vi "Main Tclk.vi"() -> ()   [LabVIEW 2018] (continued)
                        n2265 = local read "BD2 high limit array"() -> (w8137:sgl[])
                        n2266 = local read "Milling I high limit array"() -> (w8134:sgl[])
                        n2267 = local read "BD1 low limit array"() -> (w8112:sgl[])
                        n2268 = local read "BD2 low limit array"() -> (w8138:sgl[])
                        n2269 = local read "Milling I low limit array"() -> (w8133:sgl[])
                        n2270 = Build Array (concatenate)(w8147, w8123) -> (w8146:sgl[])
                        n2271 = In Range and Coerce(upper limit=w8123, x=w8100, lower limit=w8122) -> (In Range?=w8125:bool)  [unwired: 1 out]
                        n2272 = Build Array (concatenate)(w8148, w8122) -> (w8149:sgl[])
                        n2273 = Build Array (concatenate)(w8106, w8105) -> (w8113:sgl[])
                        n2274 = In Range and Coerce(upper limit=w8105, x=w8103, lower limit=w8104) -> (In Range?=w8109:bool)  [unwired: 1 out]
                        n2275 = Build Array (concatenate)(w8112, w8104) -> (w8111:sgl[])
                        n2276 = Build Array (concatenate)(w8137, w8119) -> (w8136:sgl[])
                        n2277 = In Range and Coerce(upper limit=w8119, x=w8102, lower limit=w8118) -> (In Range?=w8121:bool)  [unwired: 1 out]
                        n2278 = Build Array (concatenate)(w8138, w8118) -> (w8139:sgl[])
                        n2279 = Build Array (concatenate)(w8134, w8115) -> (w8135:sgl[])
                        n2280 = In Range and Coerce(upper limit=w8115, x=w8101, lower limit=w8114) -> (In Range?=w8117:bool)  [unwired: 1 out]
                        n2281 = Build Array (concatenate)(w8133, w8114) -> (w8132:sgl[])
                        n2282 = Not(x=w8125) -> (.not. x?=w8124:bool)
                        n2283 = Not(x=w8109) -> (.not. x?=w8110:bool)
                        n2284 = Not(x=w8121) -> (.not. x?=w8120:bool)
                        n2285 = Not(x=w8117) -> (.not. x?=w8116:bool)
                        n2286 = local write "Specimen I high limit array"(w8146) -> ()
                        n2287 = local write "Specimen I low limit array"(w8149) -> ()
                        n2288 = local write "BD1 high limit array"(w8113) -> ()
                        n2289 = local write "BD2 high limit array"(w8136) -> ()
                        n2290 = local write "Milling I high limit array"(w8135) -> ()
                        n2291 = local write "BD1 low limit array"(w8111) -> ()
                        n2292 = local write "BD2 low limit array"(w8139) -> ()
                        n2293 = local write "Milling I low limit array"(w8132) -> ()
                        n2294 = local write "Specimen I out of bound"(w8124) -> ()
                        n2295 = local write "BD1 out of bound"(w8110) -> ()
                        n2296 = local write "BD2 out of bound"(w8120) -> ()
                        n2297 = local write "Milling I out of bound"(w8116) -> ()
                      }
                      frame 2 {
                        n2298 = local read "Specimen I array"() -> (w8208:sgl[])
                        n2299 = local read "Specimen I (nA)"() -> (w8156:sgl)
                        n2300 = local read "Beam Dump 1 array"() -> (w8195:sgl[])
                        n2301 = local read "Beam Dump 1 (nA)"() -> (w8159:sgl)
                        n2302 = local read "Beam Dump 2 (nA)"() -> (w8165:sgl)
                        n2303 = local read "Milling I array"() -> (w8185:sgl[])
                        n2304 = local read "Milling I (nA)"() -> (w8164:sgl)
                        n2305 = call "Auto limits.vi"("Minimum half range"=0.5, "# of interquartile range or stdev"=6.0 ("# of sigma"), "Length"=100, "Input array"=w8208) -> ("Low limit"=w8206:dbl, "High limit"=w8207:dbl)  [unwired: 5 in, 1 out]
                        n2306 = call "Auto limits.vi"("Minimum half range"=0.5, "# of interquartile range or stdev"=6.0 ("# of sigma"), "Length"=100, "Input array"=w8195) -> ("Low limit"=w8197:dbl, "High limit"=w8196:dbl)  [unwired: 5 in, 1 out]
                        n2307 = call "Auto limits.vi"("Minimum half range"=0.5, "# of interquartile range or stdev"=6.0 ("# of sigma"), "Length"=100, "Input array"=w8185) -> ("Low limit"=w8187:dbl, "High limit"=w8186:dbl)  [unwired: 5 in, 1 out]
                        n2308 = To Single Precision Float(number=w8207) -> (single precision float=w8158:sgl)
                        n2309 = To Single Precision Float(number=w8206) -> (single precision float=w8157:sgl)
                        n2310 = To Single Precision Float(number=w8196) -> (single precision float=w8161:sgl)
                        n2311 = To Single Precision Float(number=w8197) -> (single precision float=w8160:sgl)
                        n2312 = To Single Precision Float(number=w8167) -> (single precision float=w8169:sgl)
                        n2313 = To Single Precision Float(number=w8166) -> (single precision float=w8168:sgl)
                        n2314 = To Single Precision Float(number=w8186) -> (single precision float=w8163:sgl)
                        n2315 = To Single Precision Float(number=w8187) -> (single precision float=w8162:sgl)
                        n2316 = local read "Specimen I high limit array"() -> (w8203:sgl[])
                        n2317 = local read "Specimen I low limit array"() -> (w8204:sgl[])
                        n2318 = local read "BD1 high limit array"() -> (w8200:sgl[])
                        n2319 = local read "BD2 high limit array"() -> (w8173:sgl[])
                        n2320 = local read "Milling I high limit array"() -> (w8190:sgl[])
                        n2321 = local read "BD1 low limit array"() -> (w8199:sgl[])
                        n2322 = local read "BD2 low limit array"() -> (w8174:sgl[])
                        n2323 = local read "Milling I low limit array"() -> (w8189:sgl[])
                        n2324 = Build Array (concatenate)(w8203, w8158) -> (w8202:sgl[])
                        n2325 = In Range and Coerce(upper limit=w8158, x=w8156, lower limit=w8157) -> (In Range?=w8181:bool)  [unwired: 1 out]
                        n2326 = Build Array (concatenate)(w8204, w8157) -> (w8205:sgl[])
                        n2327 = Build Array (concatenate)(w8200, w8161) -> (w8201:sgl[])
                        n2328 = In Range and Coerce(upper limit=w8161, x=w8159, lower limit=w8160) -> (In Range?=w8178:bool)  [unwired: 1 out]
                        n2329 = Build Array (concatenate)(w8199, w8160) -> (w8198:sgl[])
                        n2330 = Build Array (concatenate)(w8173, w8169) -> (w8172:sgl[])
                        n2331 = In Range and Coerce(upper limit=w8169, x=w8165, lower limit=w8168) -> (In Range?=w8171:bool)  [unwired: 1 out]
                        n2332 = Build Array (concatenate)(w8174, w8168) -> (w8175:sgl[])
                        n2333 = Build Array (concatenate)(w8190, w8163) -> (w8191:sgl[])
                        n2334 = In Range and Coerce(upper limit=w8163, x=w8164, lower limit=w8162) -> (In Range?=w8177:bool)  [unwired: 1 out]
                        n2335 = Build Array (concatenate)(w8189, w8162) -> (w8188:sgl[])
                        n2336 = Not(x=w8181) -> (.not. x?=w8180:bool)
                        n2337 = Not(x=w8178) -> (.not. x?=w8179:bool)
                        n2338 = Not(x=w8171) -> (.not. x?=w8170:bool)
                        n2339 = Not(x=w8177) -> (.not. x?=w8176:bool)
                        n2340 = local write "Specimen I high limit array"(w8202) -> ()
                        n2341 = local write "Specimen I low limit array"(w8205) -> ()
                        n2342 = local write "BD1 high limit array"(w8201) -> ()
                        n2343 = local write "BD2 high limit array"(w8172) -> ()
                        n2344 = local write "Milling I high limit array"(w8191) -> ()
                        n2345 = local write "BD1 low limit array"(w8198) -> ()
                        n2346 = local write "BD2 low limit array"(w8175) -> ()
                        n2347 = local write "Milling I low limit array"(w8188) -> ()
                        n2348 = local write "Specimen I out of bound"(w8180) -> ()
                        n2349 = local write "BD1 out of bound"(w8179) -> ()
                        n2350 = local write "BD2 out of bound"(w8170) -> ()
                        n2351 = local write "Milling I out of bound"(w8176) -> ()
                      }
                      frame 3 {
                        n2352 = local read "Specimen I array"() -> (w8267:sgl[])
                        n2353 = local read "Specimen I (nA)"() -> (w8241:sgl)
                        n2354 = local read "Beam Dump 1 array"() -> (w8254:sgl[])
                        n2355 = local read "Beam Dump 1 (nA)"() -> (w8219:sgl)
                        n2356 = local read "Beam Dump 2 array"() -> (w8251:sgl[])
                        n2357 = local read "Beam Dump 2 (nA)"() -> (w8237:sgl)
                        n2358 = local read "Milling I (nA)"() -> (w8224:sgl)
                        n2359 = expression code="X*6"(w8212) -> (w8218:sgl)
                        n2360 = expression code="X*0.5"(w8212) -> (w8217:sgl)
                        n2361 = expression code="X*6"(w8212) -> (w8214:sgl)
                        n2362 = expression code="X*0.5"(w8212) -> (w8213:sgl)
                        n2363 = expression code="X*3"(w8212) -> (w8216:sgl)
                        n2364 = expression code="X*0.2"(w8212) -> (w8215:sgl)
                        n2365 = call "Auto limits.vi"("Minimum half range"=w8217, "# of interquartile range or stdev"=w8218, "Length"=100, "Input array"=w8267) -> ("Low limit"=w8265:dbl, "High limit"=w8266:dbl)  [unwired: 5 in, 1 out]
                        n2366 = call "Auto limits.vi"("Minimum half range"=w8213, "# of interquartile range or stdev"=w8214, "Length"=100, "Input array"=w8254) -> ("Low limit"=w8256:dbl, "High limit"=w8255:dbl)  [unwired: 5 in, 1 out]
                        n2367 = call "Auto limits.vi"("Minimum half range"=w8215, "# of interquartile range or stdev"=w8216, "Length"=100, "Input array"=w8251) -> ("Low limit"=w8249:dbl, "High limit"=w8250:dbl)  [unwired: 5 in, 1 out]
                        n2368 = To Single Precision Float(number=w8266) -> (single precision float=w8243:sgl)
                        n2369 = To Single Precision Float(number=w8265) -> (single precision float=w8242:sgl)
                        n2370 = To Single Precision Float(number=w8255) -> (single precision float=w8221:sgl)
                        n2371 = To Single Precision Float(number=w8256) -> (single precision float=w8220:sgl)
                        n2372 = To Single Precision Float(number=w8250) -> (single precision float=w8239:sgl)
                        n2373 = To Single Precision Float(number=w8249) -> (single precision float=w8238:sgl)
                        n2374 = To Single Precision Float(number=w8231) -> (single precision float=w8226:sgl)
                        n2375 = To Single Precision Float(number=w8230) -> (single precision float=w8225:sgl)
                        n2376 = local read "Specimen I high limit array"() -> (w8262:sgl[])
                        n2377 = local read "Specimen I low limit array"() -> (w8263:sgl[])
                        n2378 = local read "BD1 high limit array"() -> (w8259:sgl[])
                        n2379 = local read "BD2 high limit array"() -> (w8246:sgl[])
                        n2380 = local read "BD2 low limit array"() -> (w8247:sgl[])
                        n2381 = local read "Milling I high limit array"() -> (w8235:sgl[])
                        n2382 = local read "BD1 low limit array"() -> (w8258:sgl[])
                        n2383 = local read "Milling I low limit array"() -> (w8234:sgl[])
                        n2384 = Build Array (concatenate)(w8247, w8238) -> (w8248:sgl[])
                        n2385 = Build Array (concatenate)(w8262, w8243) -> (w8261:sgl[])
                        n2386 = In Range and Coerce(upper limit=w8243, x=w8241, lower limit=w8242) -> (In Range?=w8244:bool)  [unwired: 1 out]
                        n2387 = Build Array (concatenate)(w8263, w8242) -> (w8264:sgl[])
                        n2388 = Build Array (concatenate)(w8259, w8221) -> (w8260:sgl[])
                        n2389 = In Range and Coerce(upper limit=w8221, x=w8219, lower limit=w8220) -> (In Range?=w8222:bool)  [unwired: 1 out]
                        n2390 = Build Array (concatenate)(w8258, w8220) -> (w8257:sgl[])
                        n2391 = Build Array (concatenate)(w8246, w8239) -> (w8245:sgl[])
                        n2392 = In Range and Coerce(upper limit=w8239, x=w8237, lower limit=w8238) -> (In Range?=w8240:bool)  [unwired: 1 out]
                        n2393 = Build Array (concatenate)(w8235, w8226) -> (w8236:sgl[])
                        n2394 = In Range and Coerce(upper limit=w8226, x=w8224, lower limit=w8225) -> (In Range?=w8232:bool)  [unwired: 1 out]
                        n2395 = Build Array (concatenate)(w8234, w8225) -> (w8233:sgl[])
                        n2396 = Not(x=w8244) -> (.not. x?=w8229:bool)
                        n2397 = Not(x=w8222) -> (.not. x?=w8223:bool)
                        n2398 = Not(x=w8240) -> (.not. x?=w8228:bool)
                        n2399 = Not(x=w8232) -> (.not. x?=w8227:bool)
                        n2400 = local write "Specimen I high limit array"(w8261) -> ()
                        n2401 = local write "Specimen I low limit array"(w8264) -> ()
                        n2402 = local write "BD1 high limit array"(w8260) -> ()
                        n2403 = local write "BD2 high limit array"(w8245) -> ()
                        n2404 = local write "BD2 low limit array"(w8248) -> ()
                        n2405 = local write "Milling I high limit array"(w8236) -> ()
                        n2406 = local write "BD1 low limit array"(w8257) -> ()
                        n2407 = local write "Milling I low limit array"(w8233) -> ()
                        n2408 = local write "Specimen I out of bound"(w8229) -> ()
                        n2409 = local write "BD1 out of bound"(w8223) -> ()
                        n2410 = local write "BD2 out of bound"(w8228) -> ()
                        n2411 = local write "Milling I out of bound"(w8227) -> ()
                      }
                      frame 100, Default {
                        n2412 = local read "Specimen I array"() -> (w8313:sgl[])
                        n2413 = local read "Beam Dump 1 array"() -> (w8296:sgl[])
                        n2414 = local read "Beam Dump 2 array"() -> (w8289:sgl[])
                        n2415 = local read "Milling I array"() -> (w8272:sgl[])
                        n2416 = call "Auto limits.vi"("Minimum half range"=0.5, "# of interquartile range or stdev"=6.0 ("# of sigma"), "Length"=100, "Input array"=w8313) -> ("Low limit"=w8311:dbl, "High limit"=w8312:dbl)  [unwired: 5 in, 1 out]
                        n2417 = call "Auto limits.vi"("Minimum half range"=0.5, "# of interquartile range or stdev"=6.0 ("# of sigma"), "Length"=100, "Input array"=w8296) -> ("Low limit"=w8298:dbl, "High limit"=w8297:dbl)  [unwired: 5 in, 1 out]
                        n2418 = call "Auto limits.vi"("Minimum half range"=0.5, "# of interquartile range or stdev"=6.0 ("# of sigma"), "Length"=100, "Input array"=w8289) -> ("Low limit"=w8287:dbl, "High limit"=w8288:dbl)  [unwired: 5 in, 1 out]
                        n2419 = call "Auto limits.vi"("Minimum half range"=0.5, "# of interquartile range or stdev"=6.0 ("# of sigma"), "Length"=100, "Input array"=w8272) -> ("Low limit"=w8274:dbl, "High limit"=w8273:dbl)  [unwired: 5 in, 1 out]
                        n2420 = To Single Precision Float(number=w8312) -> (single precision float=w8306:sgl)
                        n2421 = To Single Precision Float(number=w8311) -> (single precision float=w8305:sgl)
                        n2422 = To Single Precision Float(number=w8297) -> (single precision float=w8303:sgl)
                        n2423 = To Single Precision Float(number=w8298) -> (single precision float=w8304:sgl)
                        n2424 = To Single Precision Float(number=w8288) -> (single precision float=w8282:sgl)
                        n2425 = To Single Precision Float(number=w8287) -> (single precision float=w8281:sgl)
                        n2426 = To Single Precision Float(number=w8273) -> (single precision float=w8279:sgl)
                        n2427 = To Single Precision Float(number=w8274) -> (single precision float=w8280:sgl)
                        n2428 = local read "Specimen I high limit array"() -> (w8308:sgl[])
                        n2429 = local read "Specimen I low limit array"() -> (w8309:sgl[])
                        n2430 = local read "BD1 high limit array"() -> (w8301:sgl[])
                        n2431 = local read "BD2 high limit array"() -> (w8284:sgl[])
                        n2432 = local read "Milling I high limit array"() -> (w8277:sgl[])
                        n2433 = local read "BD1 low limit array"() -> (w8300:sgl[])
                        n2434 = local read "BD2 low limit array"() -> (w8285:sgl[])
                        n2435 = local read "Milling I low limit array"() -> (w8276:sgl[])
                        n2436 = Build Array (concatenate)(w8308, w8306) -> (w8307:sgl[])
                        n2437 = Build Array (concatenate)(w8309, w8305) -> (w8310:sgl[])
                        n2438 = Build Array (concatenate)(w8301, w8303) -> (w8302:sgl[])
                        n2439 = Build Array (concatenate)(w8300, w8304) -> (w8299:sgl[])
                        n2440 = Build Array (concatenate)(w8284, w8282) -> (w8283:sgl[])
                        n2441 = Build Array (concatenate)(w8285, w8281) -> (w8286:sgl[])
                        n2442 = Build Array (concatenate)(w8277, w8279) -> (w8278:sgl[])
                        n2443 = Build Array (concatenate)(w8276, w8280) -> (w8275:sgl[])
                        n2444 = local write "Specimen I high limit array"(w8307) -> ()
                        n2445 = local write "Specimen I low limit array"(w8310) -> ()
                        n2446 = local write "BD1 high limit array"(w8302) -> ()
                        n2447 = local write "BD2 high limit array"(w8283) -> ()
                        n2448 = local write "Milling I high limit array"(w8278) -> ()
                        n2449 = local write "BD1 low limit array"(w8299) -> ()
                        n2450 = local write "BD2 low limit array"(w8286) -> ()
                        n2451 = local write "Milling I low limit array"(w8275) -> ()
                      }
                    }
                  }
                }
                n2452 = local read "Delta X array for stop limit"() -> (w7979:sgl[])
                n2453 = local read "Delta Y array for stop limit"() -> (w7976:sgl[])
                n2454 = local read "X shift (nm/image)"() -> (w7965:sgl)
                n2455 = local read "Y shift (nm/image)"() -> (w7962:sgl)
                n2456 = Absolute Value(x=w7979) -> (abs(x)=w7972:sgl[])
                n2457 = Absolute Value(x=w7976) -> (abs(x)=w7971:sgl[])
                n2458 = local read "Delta X stop limit array"() -> (w7980:sgl[])
                n2459 = local read "Delta Y stop limit array"() -> (w7974:sgl[])
                n2460 = call "Auto limits.vi"("Method"="mean & stdev", "Minimum half range"=10.0 ("# of sigma"), "# of interquartile range or stdev"=6.0 ("# of sigma"), "Length"=10, "Input array"=w7972) -> ("High limit"=w7959:dbl)  [unwired: 4 in, 2 out]
                n2461 = call "Auto limits.vi"("Method"="mean & stdev", "Minimum half range"=10.0 ("# of sigma"), "# of interquartile range or stdev"=6.0 ("# of sigma"), "Length"=100, "Input array"=w7971) -> ("High limit"=w7975:dbl)  [unwired: 4 in, 2 out]
                n2462 = To Single Precision Float(number=w7959) -> (single precision float=w7982:sgl)
                n2463 = To Single Precision Float(number=w7975) -> (single precision float=w7961:sgl)
                n2464 = Absolute Value(x=w7965) -> (abs(x)=w7957:sgl)
                n2465 = Absolute Value(x=w7962) -> (abs(x)=w7958:sgl)
                n2466 = Add(x=w7982, y=w7957) -> (x+y=w7966:sgl)
                n2467 = Add(x=w7961, y=w7958) -> (x+y=w7963:sgl)
                n2468 = Build Array (concatenate)(w7980, w7966) -> (w7981:sgl[])
                n2469 = Build Array (concatenate)(w7974, w7963) -> (w7973:sgl[])
                n2470 = local write "Delta X stop limit array"(w7981) -> ()
                n2471 = local write "Delta Y stop limit array"(w7973) -> ()
              }
              frame #27 {
                n2472 = local read "Pause for reheat"() -> (w8349:bool)
                n2473 = local read "Auto re-engage"() -> (w8348:bool)
                n2474 = case shown="True" w8349 {
                  tunnel: w8348 -> [_ w8358]
                  frame False {
                  }
                  frame True {
                    n2475 = case shown="False" w8358 {
                      frame False {
                        n2476 = stacked-sequence {
                          frame #0 {
                            n2477 = local read "3D FIB-SEM Files"() -> (w8364:path)
                            n2478 = local read "Re-engage Files"() -> (w8367:path)
                            n2479 = Build Path(base path=w8364, name or relative path="LG low res.png " ("command line")) -> (appended path=w8363:path)
                            n2480 = Build Path(base path=w8367, name or relative path="pre.png " ("command line")) -> (appended path=w8362:path)
                            n2481 = Copy(9:TRUE ("run minimized? (F)"), 10:w8362, 11:w8363) -> ()  [unwired: 2 in, 3 out]
                          }
                          frame #1 {
                            n2482 = shared-variable ".\\Zeiss Library.lvlib\\Timestamp"() -> (→"Pre-reheat time":timestamp)  [unwired: 1 in, 1 out]
                            n2483 = local read "Last good FI"() -> (→"Pre-reheat FI":sgl)
                          }
                          frame #2 {
                            n2484 = local read "SEM Scan Parameters"() -> (w8370:T26)
                            n2485 = Unbundle By Name(w8370) -> ("X center (um)"=→"Pre-reheat X center (um)":sgl, "Y center (um)"=→"Pre-reheat Y center (um)":sgl, "Y stig"=w8373:sgl[][])
                            n2486 = local write "Pre-reheat Y stig"(w8373) -> ()
                          }
                        }
                      }
                      frame True {
                      }
                    }
                    n2487 = local write "Mill Manual Pause"(TRUE ("Mill Stop")) -> ()
                    n2488 = property on="Mill Manual Pause" class="Bool (strict)"("DisabledEnum"=T44."Disabled and Grayed Out" ("Disabled")) -> ()  [unwired: 2 in, 2 out]
                  }
                }
                n2489 = local read "Remaining X shift frames"() -> (w8347:u32)
                n2490 = local read "Remaining Y shift frames"() -> (w8342:u32)
                n2491 = Greater Than 0?(x=w8347) -> (x > 0?=w8346:bool)
                n2492 = Greater Than 0?(x=w8342) -> (x > 0?=w8343:bool)
                n2493 = case shown="False" w8346 {
                  tunnel: w8347 -> [_ w8357]
                  tunnel: [u32 0 w8356] -> w8345
                  frame False {
                    n2494 = local write "X shift (nm/image)"(sgl 0.0 ("X shift (nm/image)")) -> ()
                  }
                  frame True {
                    n2495 = Decrement(x=w8357) -> (x-1=w8356:u32)
                  }
                }
                n2496 = case shown="False" w8343 {
                  tunnel: w8342 -> [_ w8353]
                  tunnel: [u32 0 w8352] -> w8344
                  frame False {
                    n2497 = local write "Y shift (nm/image)"(sgl 0.0 ("X shift (nm/image)")) -> ()
                  }
                  frame True {
                    n2498 = Decrement(x=w8353) -> (x-1=w8352:u32)
                  }
                }
                n2499 = local write "Remaining X shift frames"(w8345) -> ()
                n2500 = local write "Remaining Y shift frames"(w8344) -> ()
              }
              frame #28 {
                n2501 = local read "FIB"() -> (w8382:bool)
                n2502 = local read "Alert Settings"() -> (w8380:T36)
                n2503 = local read "Log time array"() -> (w8375:u32[])
                n2504 = case shown="True" w8382 {
                  frame False {
                  }
                  frame True {
                    n2505 = local read "Temp (F)"() -> (w8419:sgl)
                    n2506 = local read "Faraday Cup (nA)"() -> (w8420:sgl)
                    n2507 = local read "Specimen I (nA)"() -> (w8421:sgl)
                    n2508 = local read "Beam Dump 1 (nA)"() -> (w8422:sgl)
                    n2509 = local read "Beam Dump 2 (nA)"() -> (w8413:sgl)
                    n2510 = local read "Milling I (nA)"() -> (w8412:sgl)
                    n2511 = local read "SEM Specimen I"() -> (w8410:dbl)
                    n2512 = local read "Milling Z voltage (V)"() -> (w8411:sgl)
                    n2513 = local read "File Information"() -> (w8423:T31)
                    n2514 = shared-variable ".\\Zeiss Library.lvlib\\Timestamp"() -> (w8416:timestamp)  [unwired: 1 in, 1 out]
                    n2515 = Unbundle By Name(w8423) -> ("File path"=w8414:path)
                    n2516 = Build Array(w8419, w8420, w8421, w8422, w8413, w8412, w8410, w8411) -> (w8417:dbl[])
                    n2517 = for {
                      tunnel: w8417 -> [w8425] mode=indexing
                      tunnel: [w8424] -> w8418 mode=indexing
                      n2518 = Format Into String(w8425) -> (resulting string=w8424:string)  [unwired: 3 in, 1 out]
                    }
                    n2519 = call "YMD log files.vi"("Input text array"=w8418, "Start new line"=FALSE, "current time"=w8416, "Log file path"=w8414) -> ()  [unwired: 8 in]
                  }
                }
                n2520 = Unbundle By Name(w8380) -> ("Focus index low limit"=w8379:sgl)
                n2521 = Array Size(array=w8375) -> (size(s)=w8374:i32)
                n2522 = local read "Focus Index"() -> (w8377:sgl)
                n2523 = Greater Than 0?(x=w8374) -> (x > 0?=w8376:bool)
                n2524 = case shown="True" w8376 {
                  tunnel: w8375 -> [_ w8397]
                  frame False {
                    w8383 = T44."Disabled and Grayed Out" ("Disabled")
                    n2525 = property on="Actual cycle time (s)" class="DigNum (strict)"("DisabledEnum"=w8383) -> ()  [unwired: 2 in, 2 out]
                    n2526 = property on="Median cycle time (s)" class="DigNum (strict)"("DisabledEnum"=w8383) -> ()  [unwired: 2 in, 2 out]
                    n2527 = property on="Daily Z removal (um)" class="DigNum (strict)"("DisabledEnum"=w8383) -> ()  [unwired: 2 in, 2 out]
                    n2528 = property on="Median cycle time est offset (s)" class="DigNum (strict)"("DisabledEnum"=w8383) -> ()  [unwired: 2 in, 2 out]
                  }
                  frame True {
                    w8387 = T44."Enabled" ("Disabled")
                    n2529 = local read "Cycle time array"() -> (w8398:u32[])
                    n2530 = shared-variable ".\\Zeiss Library.lvlib\\Timestamp"() -> (w8396:timestamp)  [unwired: 1 in, 1 out]
                    n2531 = Reverse 1D Array(array=w8397) -> (reversed array=w8401:u32[])
                    n2532 = local read "Est. cycle time (s)"() -> (w8385:u32)
                    n2533 = local read "Cycle time est offset array"() -> (w8390:i16[])
                    n2534 = Index Array(array=w8401, index=0) -> (element=w8399:u32)
                    n2535 = To Unsigned Long Integer(number=w8396) -> (unsigned 32bit integer=w8395:u32)
                    n2536 = Subtract(x=w8395, y=w8399) -> (x-y=w8392:u32)
                    "Actual cycle time (s)" <- w8392
                    n2537 = To Word Integer(number=w8385) -> (16bit integer=w8384:i16)
                    n2538 = To Word Integer(number=w8392) -> (16bit integer=w8386:i16)
                    n2539 = Build Array (concatenate)(w8398, w8392) -> (w8394:u32[])
                    n2540 = Subtract(x=w8386, y=w8384) -> (x-y=w8391:i16)
                    n2541 = local write "Cycle time array"(w8394) -> ()
                    n2542 = Build Array (concatenate)(w8390, w8391) -> (w8389:i16[])
                    n2543 = local write "Cycle time est offset array"(w8389) -> ()
                    n2544 = call <vilib>:"Median.vi"("X"=w8389) -> ("median"=→"Median cycle time est offset (s)":dbl)  [unwired: 1 out]
                    n2545 = call <vilib>:"Median.vi"("X"=w8394) -> ("median"=→"Median cycle time (s)":dbl)  [unwired: 1 out]
                    n2546 = property on="Actual cycle time (s)" class="DigNum (strict)"("DisabledEnum"=w8387) -> ()  [unwired: 2 in, 2 out]
                    n2547 = property on="Median cycle time (s)" class="DigNum (strict)"("DisabledEnum"=w8387) -> ()  [unwired: 2 in, 2 out]
                    n2548 = property on="Daily Z removal (um)" class="DigNum (strict)"("DisabledEnum"=w8387) -> ()  [unwired: 2 in, 2 out]
                    n2549 = property on="Median cycle time est offset (s)" class="DigNum (strict)"("DisabledEnum"=w8387) -> ()  [unwired: 2 in, 2 out]
                  }
                }
                n2550 = Greater Or Equal?(x=w8377, y=w8379) -> (x >= y?=w8378:bool)
                n2551 = case shown="True" w8378 {
                  frame False {
                  }
                  frame True {
                    n2552 = local read "3D FIB-SEM Files"() -> (w8405:path)
                    n2553 = Build Path(base path=w8405, name or relative path="Low res.png") -> (appended path=w8404:path)
                    n2554 = Build Path(base path=w8405, name or relative path="LG low res.png") -> (appended path=w8403:path)
                    n2555 = Copy(9:TRUE ("overwrite (F)"), 10:w8403, 11:w8404) -> ()  [unwired: 2 in, 3 out]
                  }
                }
                n2556 = local read "Reheat from last"() -> (w8381:bool)
                n2557 = case shown="True" w8381 {
                  frame False {
                  }
                  frame True {
                    w8408 = TRUE ("Mill Stop")
                    n2558 = local write "Pause for reheat"(w8408) -> ()
                    n2559 = local write "Mill Manual Pause"(w8408) -> ()
                    n2560 = property on="Mill Manual Pause" class="Bool (strict)"("DisabledEnum"=T44."Disabled and Grayed Out" ("Disabled")) -> ()  [unwired: 2 in, 2 out]
                  }
                }
              }
              frame #29 {
                n2561 = local read "Alert Settings"() -> (w8444:T36)
                n2562 = Unbundle By Name(w8444) -> ("Low limit (F)"=w8443:sgl, "High limit (F)"=w8442:sgl)
                n2563 = stacked-sequence {
                  tunnel: w8443 -> [_ w8545 _]
                  tunnel: w8442 -> [_ w8544 _]
                  tunnel: [w8482 _ _] -> w8428
                  frame #0 {
                    n2564 = local read "Log time array"() -> (w8490:u32[])
                    n2565 = shared-variable ".\\Zeiss Library.lvlib\\Timestamp"() -> (w8521:timestamp)  [unwired: 1 in, 1 out]
                    n2566 = local read "Temp array"() -> (w8520:sgl[])
                    n2567 = local read "Temp low limit array"() -> (w8503:sgl[])
                    n2568 = local read "Faraday Cup array"() -> (w8522:sgl[])
                    n2569 = local read "Faraday Cup high limit array"() -> (w8495:sgl[])
                    n2570 = local read "Faraday Cup low limit array"() -> (w8496:sgl[])
                    n2571 = local read "Specimen I high limit array"() -> (w8506:sgl[])
                    n2572 = local read "Specimen I low limit array"() -> (w8505:sgl[])
                    n2573 = local read "SEM Specimen I array"() -> (w8513:sgl[])
                    n2574 = local read "SEM Specimen I low limit array"() -> (w8501:sgl[])
                    n2575 = case shown="1" "Beam dump display" {
                      tunnel: [w8526 w8529 w8532] -> w8508
                      tunnel: [w8525 w8528 w8531] -> w8485
                      tunnel: [w8524 w8527 w8530] -> w8484
                      frame 0, Default {
                        n2576 = local read "Beam Dump 1 array"() -> (w8526:sgl[])
                        n2577 = local read "BD1 high limit array"() -> (w8525:sgl[])
                        n2578 = local read "BD1 low limit array"() -> (w8524:sgl[])
                      }
                      frame 1 {
                        n2579 = local read "Beam Dump 2 array"() -> (w8529:sgl[])
                        n2580 = local read "BD2 high limit array"() -> (w8528:sgl[])
                        n2581 = local read "BD2 low limit array"() -> (w8527:sgl[])
                      }
                      frame 2 {
                        n2582 = local read "Milling I array"() -> (w8532:sgl[])
                        n2583 = local read "Milling I high limit array"() -> (w8531:sgl[])
                        n2584 = local read "Milling I low limit array"() -> (w8530:sgl[])
                      }
                    }
                    n2585 = local read "Temp high limit array"() -> (w8504:sgl[])
                    n2586 = local read "Specimen I array"() -> (w8523:sgl[])
                    n2587 = local read "SEM Specimen I high limit array"() -> (w8502:sgl[])
                    n2588 = To Unsigned Long Integer(number=w8521) -> (unsigned 32bit integer=w8489:u32)
                    n2589 = Build Array (concatenate)(w8490, w8489) -> (w8482:u32[])
                    n2590 = Bundle(w8482, "Faraday Cup high limit array"=w8495) -> (w8493:T57)  [unwired: 1 in]
                    n2591 = Bundle(w8482, "Faraday Cup low limit array"=w8496) -> (w8494:T58)  [unwired: 1 in]
                    n2592 = Bundle(w8482, "SEM Specimen I array"=w8513) -> (w8499:cluster{u32[], "SEM Specimen I array":sgl[]})  [unwired: 1 in]
                    n2593 = Bundle(w8482, "SEM Specimen I high limit array"=w8502) -> (w8500:T59)  [unwired: 1 in]
                    n2594 = local write "Log time array"(w8482) -> ()
                    n2595 = Bundle(w8482, "Temp array"=w8520) -> (w8518:cluster{u32[], "Temp array":sgl[]})  [unwired: 1 in]
                    n2596 = Bundle(w8482, "Temp high limit array"=w8504) -> (w8519:cluster{u32[], "Temp high limit array":sgl[]})  [unwired: 1 in]
                    n2597 = Bundle(w8482, "Temp low limit array"=w8503) -> (w8517:cluster{u32[], "Temp low limit array":sgl[]})  [unwired: 1 in]
                    n2598 = Bundle(w8482, "Faraday Cup array"=w8522) -> (w8492:cluster{u32[], "Faraday Cup array":sgl[]})  [unwired: 1 in]
                    n2599 = Bundle(w8482, "Specimen I high limit array"=w8506) -> (w8511:T60)  [unwired: 1 in]
                    n2600 = Bundle(w8482, "Specimen I low limit array"=w8505) -> (w8512:T61)  [unwired: 1 in]
                    n2601 = Bundle(w8482, "SEM Specimen I low limit array"=w8501) -> (w8498:T62)  [unwired: 1 in]
                    n2602 = Bundle(w8482, "Milling I array"=w8508) -> (w8486:cluster{u32[], "Milling I array":sgl[]})  [unwired: 1 in]
                    n2603 = Bundle(w8482, "Milling I high limit array"=w8485) -> (w8488:T63)  [unwired: 1 in]
                    n2604 = Bundle(w8482, "Milling I low limit array"=w8484) -> (w8487:T64)  [unwired: 1 in]
                    n2605 = Bundle(w8482, "Specimen I array"=w8523) -> (w8510:cluster{u32[], "Specimen I array":sgl[]})  [unwired: 1 in]
                    n2606 = Build Array(w8492, w8493, w8494) -> (→"Faraday Cup log":T65)
                    n2607 = Build Array(w8518, w8519, w8517) -> (→"Temp log":cluster{u32[], "Temp low limit array":sgl[]}[])
                    n2608 = Build Array(w8510, w8511, w8512) -> (w8509:T66)
                    n2609 = Build Array(w8499, w8500, w8498) -> (w8497:T67)
                    n2610 = Build Array(w8486, w8488, w8487) -> (→"Beam Dump log":T68)
                    n2611 = Select(t=w8509, s="Specimen current toggle", f=w8497) -> (s? t:f=→"Specimen I log":T67)
                  }
                  frame #1 {
                    n2612 = local read "Delta Z mode"() -> (w8542:u8)
                    n2613 = expression code="x-0.2"(w8545) -> (w8546:sgl)
                    n2614 = expression code="x+0.2"(w8544) -> (w8547:sgl)
                    n2615 = property on="Temp log" class="XYGraph (strict)"("YScale.Minimum"=w8546) -> ()  [unwired: 2 in, 2 out]
                    n2616 = property on="Temp log" class="XYGraph (strict)"("YScale.Maximum"=w8547) -> ()  [unwired: 2 in, 2 out]
                    n2617 = case shown="0, Default" w8542 {
                      tunnel: [w8550 w8551 w8552] -> w8533
                      frame 0, Default {
                        n2618 = local read "Delta image array"() -> (w8550:sgl[])
                      }
                      frame 1 {
                        n2619 = local read "Delta Z array"() -> (w8551:sgl[])
                      }
                      frame 2 {
                        n2620 = local read "Milling Z voltage array"() -> (w8552:sgl[])
                      }
                    }
                    n2621 = Array Subset(array=w8533, index=1) -> (w8536:sgl[])  [unwired: 1 in]
                    n2622 = property on="Focus index log" class="XYGraph (strict)"() -> ("XScale.Range"=w8543:T69)  [unwired: 2 in, 2 out]
                    n2623 = Array Size(array=w8536) -> (size(s)=w8534:i32)
                    n2624 = call "Auto limits.vi"("Minimum half range"=0.2, "# of interquartile range or stdev"=3.0 ("# of sigma"), "Input array"=w8536) -> ("Low limit"=w8541:dbl, "High limit"=w8540:dbl)  [unwired: 6 in, 1 out]
                    n2625 = Not Equal To 0?(x=w8534) -> (x != 0?=w8535:bool)
                    n2626 = case shown="True" w8535 {
                      tunnel: w8540 -> [_ w8549]
                      tunnel: w8541 -> [_ w8548]
                      frame False {
                      }
                      frame True {
                        n2627 = property on="Delta Z log" class="XYGraph (strict)"("YScale.Maximum"=w8549) -> ()  [unwired: 2 in, 2 out]
                        n2628 = property on="Delta Z log" class="XYGraph (strict)"("YScale.Minimum"=w8548) -> ()  [unwired: 2 in, 2 out]
                      }
                    }
                    n2629 = property on="Delta X log" class="XYGraph (strict)"("XScale.Range"=w8543) -> ()  [unwired: 2 in, 2 out]
                    n2630 = property on="Delta Y log" class="XYGraph (strict)"("XScale.Range"=w8543) -> ()  [unwired: 2 in, 2 out]
                    n2631 = property on="Delta Z log" class="XYGraph (strict)"("XScale.Range"=w8543) -> ()  [unwired: 2 in, 2 out]
                  }
                  frame #2 {
                    w8556 = T70 {"Left"=658, "Top"=662, "Right"=1206, "Bottom"=800} ("Plot Area Bounds 3")
                    w8555 = T70 {"Left"=658, "Top"=519, "Right"=1206, "Bottom"=657} ("Plot Area Bounds 2")
                    w8554 = T70 {"Left"=658, "Top"=375, "Right"=1206, "Bottom"=513} ("Plot Area Bounds")
                    w8553 = T70 {"Left"=658, "Top"=231, "Right"=1206, "Bottom"=369} ("Plot Area Bounds")
                    n2632 = property on="Temp log" class="XYGraph (strict)"("Plot Bounds"=w8553) -> ()  [unwired: 2 in, 2 out]
                    n2633 = property on="Focus index log" class="XYGraph (strict)"("Plot Bounds"=w8553) -> ()  [unwired: 2 in, 2 out]
                    n2634 = property on="Faraday Cup log" class="XYGraph (strict)"("Plot Bounds"=w8554) -> ()  [unwired: 2 in, 2 out]
                    n2635 = property on="Delta X log" class="XYGraph (strict)"("Plot Bounds"=w8554) -> ()  [unwired: 2 in, 2 out]
                    n2636 = property on="Specimen I log" class="XYGraph (strict)"("Plot Bounds"=w8555) -> ()  [unwired: 2 in, 2 out]
                    n2637 = property on="Delta Y log" class="XYGraph (strict)"("Plot Bounds"=w8555) -> ()  [unwired: 2 in, 2 out]
                    n2638 = property on="Beam Dump log" class="XYGraph (strict)"("Plot Bounds"=w8556) -> ()  [unwired: 2 in, 2 out]
                    n2639 = property on="Delta Z log" class="XYGraph (strict)"("Plot Bounds"=w8556) -> ()  [unwired: 2 in, 2 out]
                  }
                }
                n2640 = case shown="0, Default" "Delta Z mode" {
                  tunnel: [w8479 w8480 w8481] -> w8439
                  frame 0, Default {
                    n2641 = local read "Delta image array"() -> (w8479:sgl[])
                  }
                  frame 1 {
                    n2642 = local read "Delta Z array"() -> (w8480:sgl[])
                  }
                  frame 2 {
                    n2643 = local read "Milling Z voltage array"() -> (w8481:sgl[])
                  }
                }
                n2644 = local read "Focus index array"() -> (w8429:sgl[])
                n2645 = local read "FRC array"() -> (w8427:sgl[])
                n2646 = local read "Delta X array"() -> (w8432:sgl[])
                n2647 = local read "Delta X sum array"() -> (w8431:sgl[])
                n2648 = local read "Delta Y array"() -> (w8433:sgl[])
                n2649 = local read "Delta Y sum array"() -> (w8434:sgl[])
                n2650 = case shown="False" "FI toggle" {
                  tunnel: [w8445 w8453] -> w8430
                  tunnel: w8429 -> [_ w8451]
                  tunnel: w8428 -> [w8447 w8449]
                  tunnel: w8427 -> [w8446 _]
                  frame False {
                    n2651 = Bundle(w8447, "FRC array"=w8446) -> (w8448:cluster{u32[], "FRC array":sgl[]})  [unwired: 1 in]
                    n2652 = Build Array(w8448) -> (w8445:cluster{u32[], "FRC array":sgl[]}[])
                  }
                  frame True {
                    n2653 = local read "FI low limit array"() -> (w8454:sgl[])
                    n2654 = Bundle(w8449, "Focus index array"=w8451) -> (w8450:cluster{u32[], "Focus index array":sgl[]})  [unwired: 1 in]
                    n2655 = Bundle(w8449, "FI low limit array"=w8454) -> (w8452:cluster{u32[], "FI low limit array":sgl[]})  [unwired: 1 in]
                    n2656 = Build Array(w8450, w8452) -> (w8453:cluster{u32[], "FI low limit array":sgl[]}[])
                  }
                }
                "Focus index log" <- w8430
                n2657 = case shown="False" "Delta X toggle" {
                  tunnel: [w8467 w8475] -> w8438
                  tunnel: w8432 -> [_ w8474]
                  tunnel: w8428 -> [w8469 w8473]
                  tunnel: w8431 -> [w8468 _]
                  frame False {
                    n2658 = Bundle(w8469, "Delta X sum array"=w8468) -> (w8470:cluster{u32[], "Delta X sum array":sgl[]})  [unwired: 1 in]
                    n2659 = Build Array(w8470) -> (w8467:cluster{u32[], "Delta X sum array":sgl[]}[])
                  }
                  frame True {
                    n2660 = local read "Delta X stop limit array"() -> (w8471:sgl[])
                    n2661 = Negate(x=w8471) -> (-x=w8472:sgl[])
                    n2662 = Bundle(w8473, "Delta X array"=w8474) -> (w8478:cluster{u32[], "Delta X array":sgl[]})  [unwired: 1 in]
                    n2663 = Bundle(w8473, "Delta X stop limit array"=w8471) -> (w8476:cluster{u32[], "Delta X stop limit array":sgl[]})  [unwired: 1 in]
                    n2664 = Bundle(w8473, w8472) -> (w8477:cluster{u32[], sgl[]})  [unwired: 1 in]
                    n2665 = Build Array(w8478, w8476, w8477) -> (w8475:T71)
                  }
                }
                "Delta X log" <- w8438
                n2666 = case shown="True" "Delta Y toggle" {
                  tunnel: [w8455 w8463] -> w8435
                  tunnel: w8433 -> [_ w8462]
                  tunnel: w8428 -> [w8457 w8461]
                  tunnel: w8434 -> [w8456 _]
                  frame False {
                    n2667 = Bundle(w8457, "Delta Y sum array"=w8456) -> (w8458:cluster{u32[], "Delta Y sum array":sgl[]})  [unwired: 1 in]
                    n2668 = Build Array(w8458) -> (w8455:cluster{u32[], "Delta Y sum array":sgl[]}[])
                  }
                  frame True {
                    n2669 = local read "Delta Y stop limit array"() -> (w8459:sgl[])
                    n2670 = Negate(x=w8459) -> (-x=w8460:sgl[])
                    n2671 = Bundle(w8461, "Delta Y array"=w8462) -> (w8466:cluster{u32[], "Delta Y array":sgl[]})  [unwired: 1 in]
                    n2672 = Bundle(w8461, "Delta Y stop limit array"=w8459) -> (w8464:cluster{u32[], "Delta Y stop limit array":sgl[]})  [unwired: 1 in]
                    n2673 = Bundle(w8461, w8460) -> (w8465:cluster{u32[], sgl[]})  [unwired: 1 in]
                    n2674 = Build Array(w8466, w8464, w8465) -> (w8463:T72)
                  }
                }
                "Delta Y log" <- w8435
                n2675 = Bundle(w8428, "Milling Z voltage array"=w8439) -> (→"Delta Z log":cluster{u32[], "Milling Z voltage array":sgl[]})  [unwired: 1 in]
              }
              frame #30 {
                n2676 = local read "3D FIB-SEM Files"() -> (w8557:path)
                n2677 = local read "SEM Scan Parameters"() -> (w8564:T26)
                n2678 = Unbundle By Name(w8564) -> ("Y tiles"=w8570:u8, "X tiles"=w8571:u8)
                n2679 = Decrement(x=w8570) -> (x-1=w8568:u8)
                n2680 = Decrement(x=w8571) -> (x-1=w8569:u8)
                n2681 = Format Into String(w8568) -> (resulting string=w8565:string)  [unwired: 3 in, 1 out]
                n2682 = Format Into String(w8569) -> (resulting string=w8567:string)  [unwired: 3 in, 1 out]
                n2683 = Concatenate Strings("Primary_grid_" ("name or relative path"), w8565, "-" ("name or relative path"), w8567, ".png" ("name or relative path")) -> (w8559:string)
                n2684 = Build Path(base path=w8557, name or relative path=w8559) -> (appended path=w8560:path)
                n2685 = File/Directory Info(path=w8560) -> (error out=w8561:errorcluster)  [unwired: 1 in, 6 out]
                n2686 = Unbundle By Name(w8561) -> ("status"=w8558:bool)
                n2687 = case shown="False" w8558 {
                  tunnel: w8557 -> [w8572 _]
                  frame False {
                    n2688 = local read "SEM Scan Parameters"() -> (w8575:T26)
                    n2689 = Unbundle By Name(w8575) -> ("Y tiles"=w8574:u8, "X tiles"=w8573:u8)
                    n2690 = for {
                      N: w8574 -> [_]
                      tunnel: w8572 -> [w8577]
                      tunnel: w8573 -> [w8576]
                      i -> [w8578]
                      n2691 = for {
                        N: w8576 -> [_]
                        tunnel: w8578 -> [w8587]
                        tunnel: w8577 -> [w8582]
                        i -> [w8588]
                        n2692 = Format Into String(w8587) -> (resulting string=w8591:string)  [unwired: 3 in, 1 out]
                        n2693 = Format Into String(w8588) -> (resulting string=w8593:string)  [unwired: 3 in, 1 out]
                        n2694 = Concatenate Strings(w8591, "-" ("name or relative path"), w8593, ".png" ("name or relative path")) -> (w8585:string)
                        n2695 = Concatenate Strings("Primary_grid_" ("command line"), w8585) -> (w8584:string)
                        n2696 = Concatenate Strings("post_" ("name or relative path"), w8585) -> (w8583:string)
                        n2697 = Build Path(base path=w8582, name or relative path=w8584) -> (appended path=w8580:path)
                        n2698 = Build Path(base path=w8582, name or relative path=w8583) -> (appended path=w8581:path)
                        n2699 = Move(source path=w8580, 9:TRUE ("run minimized? (F)"), 10:w8581) -> ()  [unwired: 2 in, 3 out]
                      }
                    }
                  }
                  frame True {
                  }
                }
              }
              frame #31 {
                n2700 = local read "FI grid array tiled"() -> (w8604:sgl[][][][][])
                n2701 = local read "WD array tiled"() -> (w8597:sgl[][][])
                n2702 = local read "FI array tiled"() -> (w8598:sgl[][][])
                n2703 = local read "AF Count"() -> (w8599:u8)
                n2704 = local read "AF Steps"() -> (w8601:u8)
                n2705 = local read "Skip Steps tiled"() -> (w8600:u8[][])
                n2706 = local read "Auto Focus"() -> (w8602:bool)
                n2707 = Empty Array?(array=w8597) -> (empty?=w8596:bool)
                n2708 = Not(x=w8602) -> (.not. x?=w8603:bool)
                n2709 = local read "Focus Index Options"() -> (w8595:T28)
                n2710 = Unbundle By Name(w8595) -> ("Keep aspect ratio"=w8594:bool)
                n2711 = case shown="False" w8596 {
